vi "WS1050 DVA CP Setting.vi"(8 "error in (no error)":errorcluster, 10 "DVA":bool, 11 "CP with DVA ON":i32(ring) items=["CP HDC 35V", "CP HDC 40.25V", "CP HDC 27.5V", "CP HDC 30.5V", "CP HDC 44V", "CP HDC 50V", "CP HDC 55V", "CP HDC 42.5V", "CP HDC 32V"]) -> (0 "error out":errorcluster, 3 "Data Out":string)   [LabVIEW 2012]
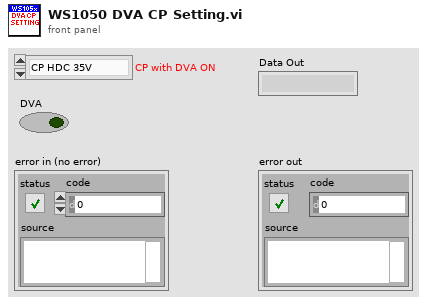
[diagram p1: front panel]
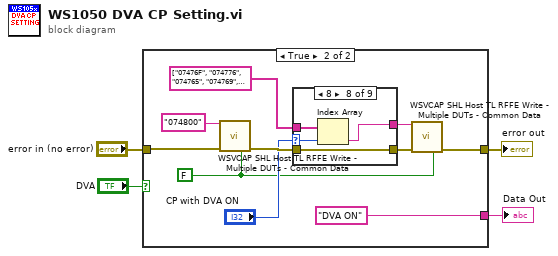
[diagram p0: block diagram]
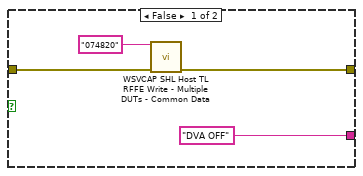
[diagram p2: hidden frame]
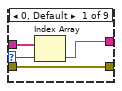
[diagram p3: hidden frame]
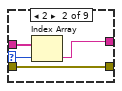
[diagram p4: hidden frame]
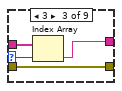
[diagram p5: hidden frame]
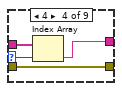
[diagram p6: hidden frame]
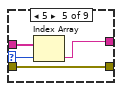
[diagram p7: hidden frame]
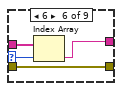
[diagram p8: hidden frame]
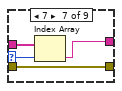
[diagram p9: hidden frame]
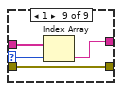
[diagram p10: hidden frame]
diagram:
  n1 = case shown="True" "DVA" {
    tunnel: "error in (no error)" -> [w8 w16]
    tunnel: [w7 w15] -> w3
    tunnel: ["DVA OFF" ("Data Out") "DVA ON" ("Data Out")] -> w2
    frame False {
      n2 = call "WSVCAP SHL Host TL RFFE Write - Multiple DUTs - Common Data.vi"("Data Out"="074820", "error in"=w8) -> ("error out"=w7:errorcluster)  [unwired: 13 in]
    }
    frame True {
      w9 = FALSE ("Log (T)")
      n3 = call "WSVCAP SHL Host TL RFFE Write - Multiple DUTs - Common Data.vi"("Data Out"="074800", "error in"=w16, "Log (T)"=w9) -> ("error out"=w14:errorcluster)  [unwired: 12 in]
      n4 = case shown="8" "CP with DVA ON" {
        selector: "CP with DVA ON" -> [w22 w26 w30 w34 w38 w42 w46 w50 w54]
        tunnel: [w21 w25 w29 w33 w37 w41 w45 w49 w52] -> w11
        tunnel: [w20 w24 w28 w32 w36 w40 w44 w48 w53] -> w13
        tunnel: w14 -> [w20 w24 w28 w32 w36 w40 w44 w48 w53]
        tunnel: string[] ["07476F", "074776", "074765", "074769", "07477B", "07477C", "07477D", "074779", "07476B"] -> [w19 w23 w27 w31 w35 w39 w43 w47 w51]
        frame 0, Default {
          n5 = Index Array(array=w19, index=w22) -> (element=w21:string)
        }
        frame 2 {
          n6 = Index Array(array=w23, index=w26) -> (element=w25:string)
        }
        frame 3 {
          n7 = Index Array(array=w27, index=w30) -> (element=w29:string)
        }
        frame 4 {
          n8 = Index Array(array=w31, index=w34) -> (element=w33:string)
        }
        frame 5 {
          n9 = Index Array(array=w35, index=w38) -> (element=w37:string)
        }
        frame 6 {
          n10 = Index Array(array=w39, index=w42) -> (element=w41:string)
        }
        frame 7 {
          n11 = Index Array(array=w43, index=w46) -> (element=w45:string)
        }
        frame 8 {
          n12 = Index Array(array=w47, index=w50) -> (element=w49:string)
        }
        frame 1 {
          n13 = Index Array(array=w51, index=w54) -> (element=w52:string)
        }
      }
      n14 = call "WSVCAP SHL Host TL RFFE Write - Multiple DUTs - Common Data.vi"("Data Out"=w11, "error in"=w13, "Log (T)"=w9) -> ("error out"=w15:errorcluster)  [unwired: 12 in]
    }
  }
  "error out" <- w3
  "Data Out" <- w2
